vi "Intensity Graph to Igor Graph.vi"(8 "error in (no error)":errorcluster, 10 "Intensity Graph Reference":refnum<vi>, 11 "Path":path=path "C:/temp") -> (0 "error out":errorcluster, 3 "file":path)   [LabVIEW 2016, in "Data.ITX.lvclass"]
uses:
  Data.ITX.lvclass
  <userlib>/LevyLab/Graph Utilities/graph_utilities.lvclass/graph_utilities.ctl
  <userlib>/LevyLab/Graph Utilities/graph_utilities.lvclass
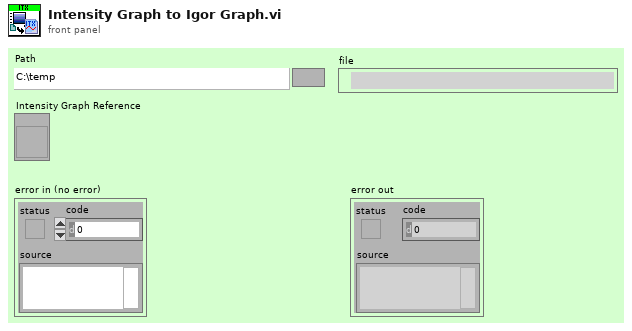
[diagram p1: front panel]
types:
  T1 = cluster{"Value":dbl[][], "X Scale":dbl[], "Y Scale":dbl[]}
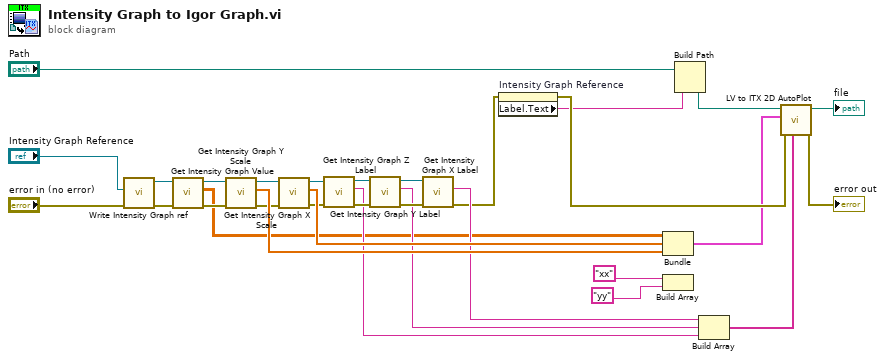
[diagram p0: block diagram]
diagram:
  n1 = call <userlib>:"Write Intensity Graph ref.vi"("error in (no error)"="error in (no error)", "Intensity Graph"="Intensity Graph Reference") -> ("error out"=w28:errorcluster, "graph_utilities out"=w29:refnum<class "graph_utilities.lvclass">)  [unwired: 8 in]
  n2 = call <userlib>:"Get Intensity Graph Value.vi"("error in (no error)"=w28, "graph_utilities in"=w29) -> ("error out"=w25:errorcluster, "Value"=w11:dbl[][], "graph_utilities out"=w26:refnum<class "graph_utilities.lvclass">)  [unwired: 7 in]
  n3 = call <userlib>:"Get Intensity Graph Y Scale.vi"("error in (no error)"=w25, "graph_utilities in"=w26) -> ("error out"=w22:errorcluster, "Y Scale"=w24:dbl[], "graph_utilities out"=w23:refnum<class "graph_utilities.lvclass">)  [unwired: 6 in, 1 out]
  n4 = call <userlib>:"Get Intensity Graph X Scale.vi"("error in (no error)"=w22, "graph_utilities in"=w23) -> ("error out"=w17:errorcluster, "X Scale"=w27:dbl[], "graph_utilities out"=w16:refnum<class "graph_utilities.lvclass">)  [unwired: 6 in, 1 out]
  n5 = call <userlib>:"Get Intensity Graph Z Label.vi"("error in (no error)"=w17, "graph_utilities in"=w16) -> ("error out"=w19:errorcluster, "Z Label"=w13:string, "graph_utilities out"=w18:refnum<class "graph_utilities.lvclass">)  [unwired: 7 in]
  n6 = call <userlib>:"Get Intensity Graph Y Label.vi"("error in (no error)"=w19, "graph_utilities in"=w18) -> ("error out"=w21:errorcluster, "Y Label"=w14:string, "graph_utilities out"=w20:refnum<class "graph_utilities.lvclass">)  [unwired: 7 in]
  n7 = call <userlib>:"Get Intensity Graph X Label.vi"("error in (no error)"=w21, "graph_utilities in"=w20) -> ("error out"=w5:errorcluster, "X Label"=w15:string)  [unwired: 7 in, 1 out]
  n8 = property on="Intensity Graph Reference" class="LVObjRef (strict)"(error in=w5) -> (error out=w4:errorcluster, "Label.Text"=w3:string)  [unwired: 1 in, 1 out]
  n9 = Bundle("Value"=w11, "X Scale"=w27, "Y Scale"=w24) -> (w1:T1)  [unwired: 1 in]
  n10 = Build Array("xx" ("X Scale.Name Label.Text"), "yy" ("X Scale.Name Label.Text")) -> ()  [unwired: 1 out]
  n11 = Build Path(base path="Path", name or relative path=w3) -> (appended path=w2:path)
  n12 = Build Array(w15, w14, w13) -> (w10:string[])
  n13 = call "LV to ITX 2D AutoPlot.vi"("X,Y,Z Labels"=w10, "error in"=w4, "2D, X, Y (Cluster)"=w1, "path"=w2) -> ("error out"=→"error out":errorcluster, "file"=→"file":path)  [unwired: 6 in]
